vi "Download and Run Installer.vi"(8 "error in (no error)":errorcluster, 10 "path to download":string, 11 "SelfUpdate in":refnum<class "SelfUpdate.lvclass">) -> (0 "error out":errorcluster, 3 "SelfUpdate out":refnum<class "SelfUpdate.lvclass">)   [LabVIEW 2019, in "SelfUpdate.lvclass"]
uses:
  SelfUpdate.lvclass
panel:
  out "concatenated string":string
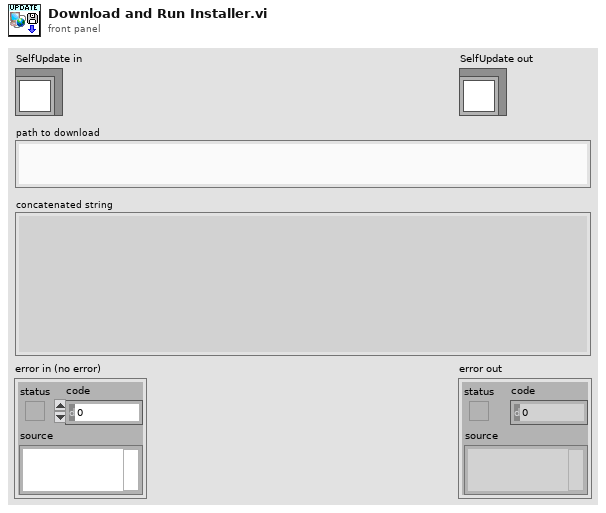
[diagram p1: front panel]
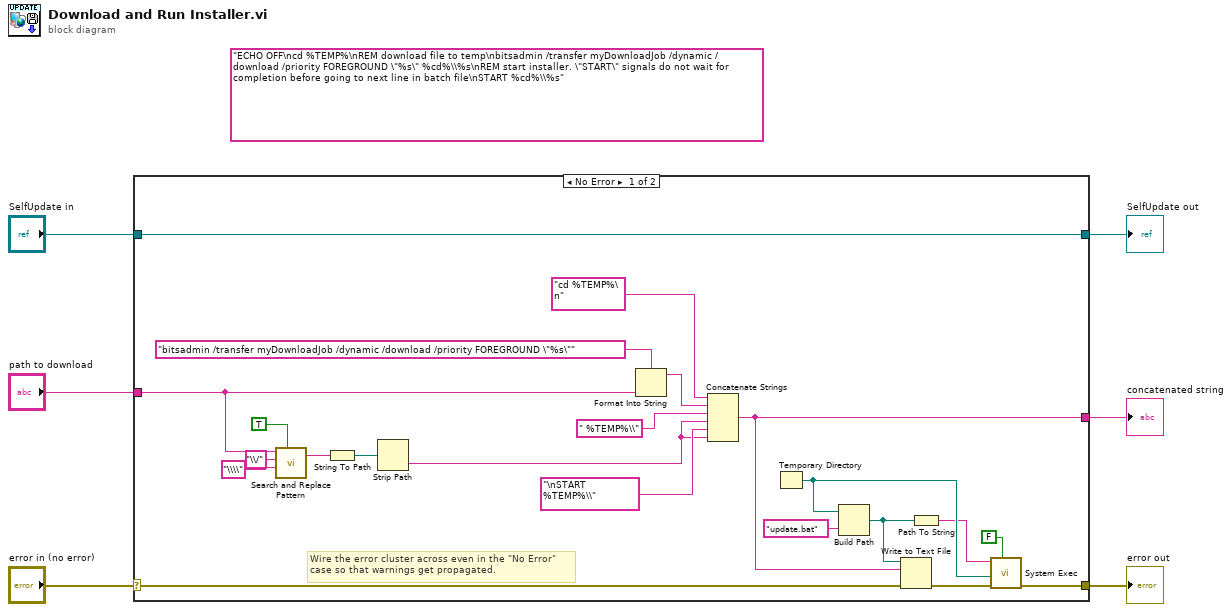
[diagram p0: block diagram]
diagram:
  (unwired) "ECHO OFF\ncd %TEMP%\nREM download file to temp\nbitsadmin /transfer myDownloadJob /dynamic /download /priority FOREGROUND \"%s\" %cd%\\%s\nREM start installer. \"START\" signals do not wait for completion before going to next line in batch file\nSTART %cd%\\%s" ("regular expression")
  n1 = case shown="No Error" "error in (no error)" {
    selector: "error in (no error)" -> [w17 w30]
    tunnel: [w12 w30] -> w5
    tunnel: [w28 w29] -> w3
    tunnel: "SelfUpdate in" -> [w28 w29]
    tunnel: "path to download" -> [w14 _]
    tunnel: [w15 _] -> w1
    frame No Error {
      # "Wire the error cluster across even in the \"No Error\"\ncase so that warnings get propagated."
      n2 = call <vilib>:"Search and Replace Pattern.vi"("string"=w14, "regular expression (\"\")"="\\/" ("regular expression (\"\")"), "replace string (\"\")"="\\\\" ("regular expression (\"\")"), "replace all? (F)"=TRUE) -> ("result string"=w23:string)  [unwired: 1 in, 1 out]
      n3 = String To Path(string=w23) -> (path=w22:path)
      n4 = Strip Path(path=w22) -> (name=w16:string)  [unwired: 1 out]
      n5 = Format Into String(format string="bitsadmin /transfer myDownloadJob /dynamic /download /priority FOREGROUND \"%s\"" ("regular expression"), w14) -> (resulting string=w21:string)  [unwired: 2 in, 1 out]
      n6 = Concatenate Strings("cd %TEMP%\n" ("regular expression"), w21, " %TEMP%\\" ("regular expression"), w16, "\nSTART %TEMP%\\" ("regular expression"), w16) -> (w15:string)
      n7 = Temporary Directory() -> (w11:path)
      n8 = Build Path(base path=w11, name or relative path="update.bat" ("prompt (Choose or enter file path)")) -> (appended path=w8:path)
      n9 = Write to Text File(file (use dialog)=w8, text=w15, error in=w17) -> (error out=w13:errorcluster)  [unwired: 1 in, 2 out]
      n10 = Path To String(path=w8) -> (string=w7:string)
      n11 = call <vilib>:"System Exec.vi"("wait until completion? (T)"=FALSE, "error in (no error)"=w13, "working directory"=w11, "command line"=w7) -> ("error out"=w12:errorcluster)  [unwired: 4 in, 3 out]
    }
    frame Error {
    }
  }
  "error out" <- w5
  "SelfUpdate out" <- w3
  "concatenated string" <- w1
